vi "R7Initialize.vi"(8 "error in (no error)":errorcluster) -> (0 "error out":errorcluster)   [LabVIEW 2016]
uses:
  Controls/pH_SetParams Standard.ctl
  Controls/R7SBR_SetParams.ctl
  Controls/pH_Manual Standard.ctl
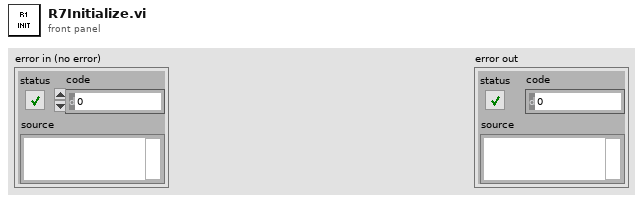
[diagram p1: front panel]
types:
  T1 = typedef "R7SBR_SetParams.ctl" = cluster{"Phase":string, "Time, min":dbl, "SBR_Manual (Standard)":cluster{"Media Pump":bool, "Water Pump":bool, "Effluent Pump":bool, "Release Valve":bool, "N2 Valve":bool, "Recirc Pump":bool}}[]
  T2 = cluster{"Set Point, mgN/L":dbl, "Tolerance, mgN/L":dbl, "Pump Gain":dbl, "Max Volume/Cycle, mL":dbl}
  T3 = cluster{"Media Pump":bool, "Water Pump":bool, "Effluent Pump":bool, "Release Valve":bool, "Gas Pump":bool, bool}
  T4 = cluster{"Set Point, mg/L":dbl, "Tolerance, mg/L":dbl, "N2 Valve Gain":dbl, "Air Valve Gain":dbl}
  T5 = typedef "pH_SetParams Standard.ctl" = cluster{"Set Point":dbl, "Tolerance":dbl, "Pump Time On, secs":dbl}
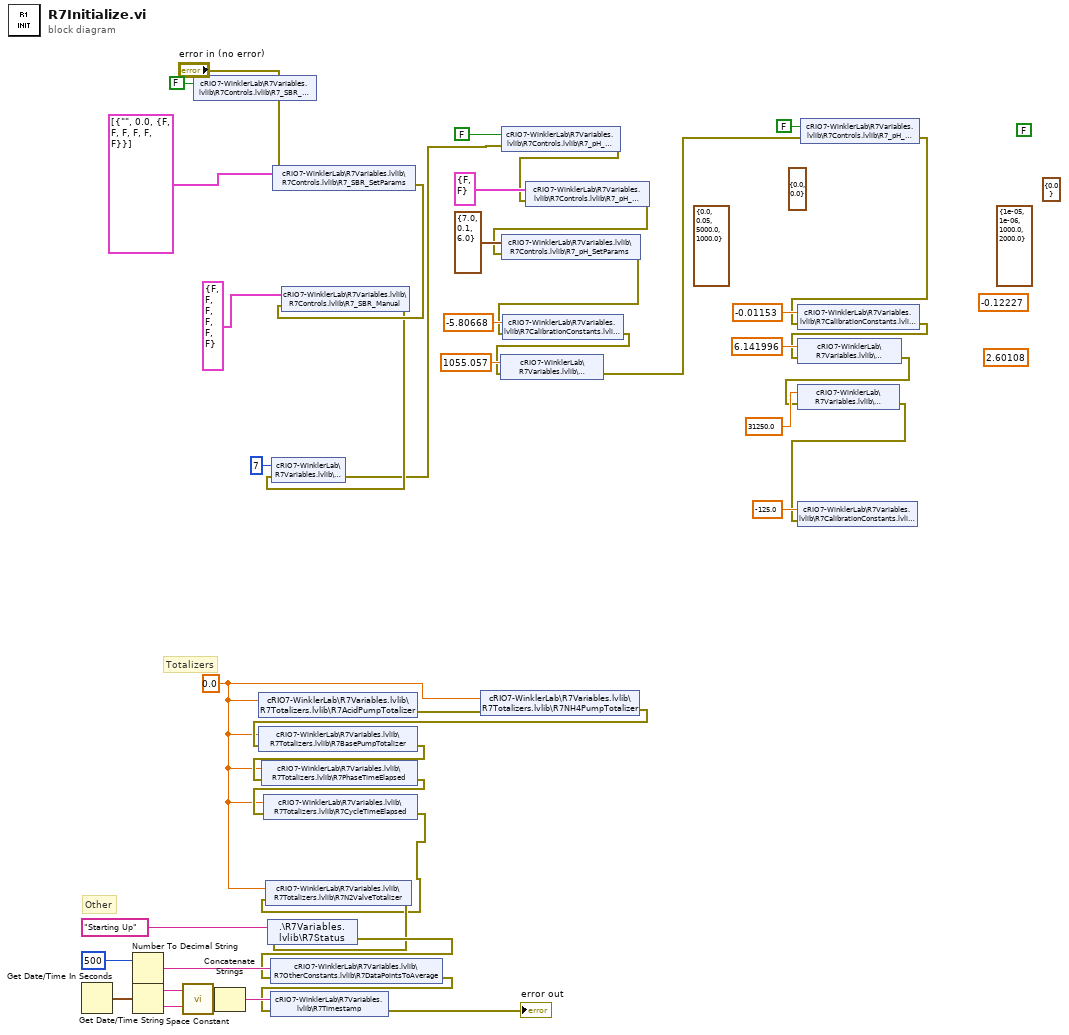
[diagram p0: block diagram]
diagram:
  (unwired) 2.60108 ("NH4PumpSlope")
  (unwired) -0.12227 ("NH4PumpIntercept")
  (unwired) T2 {"Set Point, mgN/L"=1e-05, "Tolerance, mgN/L"=1e-06, "Pump Gain"=1000.0, "Max Volume/Cycle, mL"=2000.0} ("R1_NH4_SetParams")
  (unwired) FALSE ("R1_NH4_Switch")
  (unwired) cluster{"NH4 Pump Flowrate, ml/min":dbl} {"NH4 Pump Flowrate, ml/min"=0.0} ("R1NH4Manual")
  w1 = 0.0 ("R1PhaseTimeElapsed")
  (unwired) T4 {"Set Point, mg/L"=0.0, "Tolerance, mg/L"=0.05, "N2 Valve Gain"=5000.0, "Air Valve Gain"=1000.0} ("R1DOSetParams")
  (unwired) cluster{"Air MFC":dbl, "N2 MFC":dbl} {"Air MFC"=0.0, "N2 MFC"=0.0} ("R1DOManual")
  # "Totalizers"
  # "Other"
  n1 = Get Date/Time In Seconds() -> (seconds since 1Jan1904=w21:timestamp)
  n2 = Number To Decimal String(number=500 ("R1DataPointsToAverage")) -> (decimal integer string=w36:string)  [unwired: 1 in]
  n3 = Get Date/Time String(seconds (now)=w21) -> (date string=w14:string, time string=w20:string)  [unwired: 2 in]
  n4 = call <vilib>:"Space Constant.vi"() -> ("String"=w19:string)
  n5 = shared-variable "cRIO7-WinklerLab\\R7Variables.lvlib\\R7Controls.lvlib\\R7_SBR_Switch"(FALSE ("R1SBRSwitch")) -> ()  [unwired: 1 in, 1 out]
  n6 = Concatenate Strings(w14, w19, w20) -> (w17:string)
  n7 = shared-variable "cRIO7-WinklerLab\\R7Variables.lvlib\\R7Totalizers.lvlib\\R7AcidPumpTotalizer"(w1) -> (error out=w11:errorcluster)  [unwired: 1 in]
  n8 = shared-variable "cRIO7-WinklerLab\\R7Variables.lvlib\\R7Controls.lvlib\\R7_SBR_SetParams"(T1 [{"Phase"="", "Time, min"=0.0, "SBR_Manual (Standard)"={"Media Pump"=FALSE, "Water Pump"=FALSE, "Effluent Pump"=FALSE, "Release Valve"=FALSE, "N2 Valve"=FALSE, "Recirc Pump"=FALSE}}] ("R7_SBR_SetParams"), error in="error in (no error)") -> (error out=w5:errorcluster)
  n9 = shared-variable "cRIO7-WinklerLab\\R7Variables.lvlib\\R7Controls.lvlib\\R7_SBR_Manual"(T3 {"Media Pump"=FALSE, "Water Pump"=FALSE, "Effluent Pump"=FALSE, "Release Valve"=FALSE, "Gas Pump"=FALSE, FALSE} ("R1SBRManual"), error in=w5) -> (error out=w4:errorcluster)
  n10 = shared-variable "cRIO7-WinklerLab\\R7Variables.lvlib\\R7OtherConstants.lvlib\\R7No"(i16 7 ("R1No"), error in=w4) -> (error out=w3:errorcluster)
  n11 = shared-variable "cRIO7-WinklerLab\\R7Variables.lvlib\\R7Totalizers.lvlib\\R7NH4PumpTotalizer"(w1, error in=w11) -> (error out=w12:errorcluster)
  n12 = shared-variable "cRIO7-WinklerLab\\R7Variables.lvlib\\R7Totalizers.lvlib\\R7BasePumpTotalizer"(w1, error in=w12) -> (error out=w15:errorcluster)
  n13 = shared-variable "cRIO7-WinklerLab\\R7Variables.lvlib\\R7Totalizers.lvlib\\R7PhaseTimeElapsed"(w1, error in=w15) -> (error out=w22:errorcluster)
  n14 = shared-variable "cRIO7-WinklerLab\\R7Variables.lvlib\\R7Totalizers.lvlib\\R7CycleTimeElapsed"(w1, error in=w22) -> (error out=w2:errorcluster)
  n15 = shared-variable "cRIO7-WinklerLab\\R7Variables.lvlib\\R7Totalizers.lvlib\\R7N2ValveTotalizer"(w1, error in=w2) -> (error out=w10:errorcluster)
  n16 = shared-variable ".\\R7Variables.lvlib\\R7Status"("Starting Up" ("R1Status"), error in=w10) -> (error out=w23:errorcluster)
  n17 = shared-variable "cRIO7-WinklerLab\\R7Variables.lvlib\\R7OtherConstants.lvlib\\R7DataPointsToAverage"(w36, error in=w23) -> (error out=w16:errorcluster)
  n18 = shared-variable "cRIO7-WinklerLab\\R7Variables.lvlib\\R7Timestamp"(w17, error in=w16) -> (error out=→"error out":errorcluster)
  n19 = shared-variable "cRIO7-WinklerLab\\R7Variables.lvlib\\R7Controls.lvlib\\R7_pH_Switch"(FALSE ("R1pHSwitch"), error in=w3) -> (error out=w31:errorcluster)
  n20 = shared-variable "cRIO7-WinklerLab\\R7Variables.lvlib\\R7Controls.lvlib\\R7_pH_Manual"(cluster{"Acid Pump":bool, "Base Pump":bool} {"Acid Pump"=FALSE, "Base Pump"=FALSE} ("R1pHManual"), error in=w31) -> (error out=w30:errorcluster)
  n21 = shared-variable "cRIO7-WinklerLab\\R7Variables.lvlib\\R7Controls.lvlib\\R7_pH_SetParams"(T5 {"Set Point"=7.0, "Tolerance"=0.1, "Pump Time On, secs"=6.0} ("R1pHSetParams"), error in=w30) -> (error out=w29:errorcluster)
  n22 = shared-variable "cRIO7-WinklerLab\\R7Variables.lvlib\\R7CalibrationConstants.lvlib\\R7pHIntercept"(-5.80668 ("R12pHInt"), error in=w29) -> (error out=w26:errorcluster)
  n23 = shared-variable "cRIO7-WinklerLab\\R7Variables.lvlib\\R7CalibrationConstants.lvlib\\R7pHSlope"(1055.057 ("R1pHSlope"), error in=w26) -> (error out=w27:errorcluster)
  n24 = shared-variable "cRIO7-WinklerLab\\R7Variables.lvlib\\R7Controls.lvlib\\R7_pH_Switch"(FALSE ("R1pHSwitch"), error in=w27) -> (error out=w8:errorcluster)
  n25 = shared-variable "cRIO7-WinklerLab\\R7Variables.lvlib\\R7CalibrationConstants.lvlib\\R7DOIntercept"(-0.01153 ("R1DOInt"), error in=w8) -> (error out=w25:errorcluster)
  n26 = shared-variable "cRIO7-WinklerLab\\R7Variables.lvlib\\R7CalibrationConstants.lvlib\\R7DOSlope"(6.141996 ("R1DOSlope"), error in=w25) -> (error out=w24:errorcluster)
  n27 = shared-variable "cRIO7-WinklerLab\\R7Variables.lvlib\\R7CalibrationConstants.lvlib\\R7N2Slope"(31250.0 ("R1AirSlope"), error in=w24) -> (error out=w7:errorcluster)
  n28 = shared-variable "cRIO7-WinklerLab\\R7Variables.lvlib\\R7CalibrationConstants.lvlib\\R7N2Intercept"(-125.0 ("R1N2Intercept"), error in=w7) -> ()  [unwired: 1 out]
